vi "Right Front Rocket Backup.vi"() -> (4 "path":cluster{"X":dbl, "Y":dbl}[](array[cluster])=[{"X"=200.0, "Y"=26.0}, {"X"=199.1943498032167, "Y"=26.591866844934284}, {"X"=198.38873809601802, "Y"=27.18374953225293}, {"X"=197.5831805333619, "Y"=27.775644921567796}, {"X"=196.7776935699249, "Y"=28.367551744638334}, {"X"=195.97230663271714, "Y"=28.95947685312332}, {"X"=195.16706591924, "Y"=29.551435458333945}, {"X"=194.36203025886132, "Y"=30.143446988636807}, {"X"=193.5572652684043, "Y"=30.735530675900026}, {"X"=192.75284191693686, "Y"=31.32770409196553}, {"X"=191.9488416559131, "Y"=31.919985289972765}, {"X"=191.1453662297423, "Y"=32.512397057826604}, {"X"=190.34254864947067, "Y"=33.104971168873284}, {"X"=189.54056281731533, "Y"=33.69775128282373}, {"X"=188.73963160206324, "Y"=34.29079446437416}, {"X"=187.94003519101045, "Y"=34.88417230079357}, {"X"=187.14212237118593, "Y"=35.47797290200322}, {"X"=186.34632703384437, "Y"=36.07230473652726}, {"X"=185.5531911950038, "Y"=36.667302723675775}, {"X"=184.76339581382143, "Y"=37.26313582570225}, {"X"=183.97779546937824, "Y"=37.860020685493126}, {"X"=183.1974762909218, "Y"=38.458217383512036}, {"X"=182.42378519481926, "Y"=39.058094370726934}, {"X"=181.65844307990056, "Y"=39.66003129580096}, {"X"=180.90360190480678, "Y"=40.264622933863706}, {"X"=180.16194289999132, "Y"=40.87251655708369}, {"X"=179.43687179220336, "Y"=41.484549595685024}, {"X"=178.73266346217133, "Y"=42.10181051088304}, {"X"=178.05466925868603, "Y"=42.72564542605129}, {"X"=177.40962348032767, "Y"=43.35772858802012}, {"X"=176.80601063295643, "Y"=44.000177475204424}, {"X"=176.25449894606365, "Y"=44.655669174547775}, {"X"=175.76848917552144, "Y"=45.327566980849404}, {"X"=175.36482277513522, "Y"=46.02008856392197}, {"X"=175.0646779497543, "Y"=46.73853223710994}, {"X"=174.86614653066542, "Y"=47.51051459305893}, {"X"=174.7484379619757, "Y"=48.325063754078045}, {"X"=174.6950112849843, "Y"=49.17344929096942}, {"X"=174.6927035694691, "Y"=50.04871852011999}, {"X"=174.73104103819261, "Y"=50.945330054404096}, {"X"=174.80169247736674, "Y"=51.85886492548568}, {"X"=174.89803246459678, "Y"=52.78579710225695}, {"X"=175.01479085792968, "Y"=53.72330893577166}, {"X"=175.14777214158292, "Y"=54.66914161793746}, {"X"=175.293632277303, "Y"=55.621473844165195}, {"X"=175.44970252687955, "Y"=56.578826266134335}, {"X"=175.61385096312907, "Y"=57.53997634478085}, {"X"=175.7843670904187, "Y"=58.5039152993254}, {"X"=175.95989103496223, "Y"=59.469756162119815}, {"X"=176.13929548545426, "Y"=60.43673938057879}, {"X"=176.32170057144518, "Y"=61.404155893682265}, {"X"=176.50635201235707, "Y"=62.37130891959189}, {"X"=176.6926108918171, "Y"=63.33749871042447}, {"X"=176.8799414404591, "Y"=64.30197853375324}, {"X"=177.06786159705038, "Y"=65.26390340878352}, {"X"=177.2559091660838, "Y"=66.2222899350715}, {"X"=177.44363053363736, "Y"=67.17597342387097}, {"X"=177.63056456629263, "Y"=68.12354689215407}, {"X"=177.81621186609976, "Y"=69.06328130793628}, {"X"=178.0, "Y"=69.99303135888502}], 6 "Reverse Path?":bool=TRUE)   [LabVIEW 2018]
uses:
  AutonBuilder/Typedef/Data Point.ctl
panel:
  in  "Data Points":T1[](array[typedef])=[{"X"=200.0, "Y"=26.0, "Theta"=0.0, "Speed %"=0.0, "Disabled?"=FALSE}, {"X"=173.13402061855672, "Y"=45.721254355400696, "Theta"=0.0, "Speed %"=0.0, "Disabled?"=FALSE}, {"X"=178.0, "Y"=69.99303135888502, "Theta"=0.0, "Speed %"=0.0, "Disabled?"=FALSE}]
  out "Graph":cluster{dbl[], dbl[]}[](graph)=[{[180.5, 214.0, 214.0, 180.5, 180.5], [40.25, 40.25, 11.75, 11.75, 40.25]}, {[200.0, 173.13402061855672, 178.0], [26.0, 45.721254355400696, 69.99303135888502]}, {[200.0, 199.1943498032167, 198.38873809601802, 197.5831805333619, 196.7776935699249, 195.97230663271714, 195.16706591924, 194.36203025886132, 193.5572652684043, 192.75284191693686, 191.9488416559131, 191.1453662297423, 190.34254864947067, 189.54056281731533, 188.73963160206324, 187.94003519101045, 187.14212237118593, 186.34632703384437, 185.5531911950038, 184.76339581382143, 183.97779546937824, 183.1974762909218, 182.42378519481926, 181.65844307990056, 180.90360190480678, 180.16194289999132, 179.43687179220336, 178.73266346217133, 178.05466925868603, 177.40962348032767, 176.80601063295643, 176.25449894606365, 175.76848917552144, 175.36482277513522, 175.0646779497543, 174.86614653066542, 174.7484379619757, 174.6950112849843, 174.6927035694691, 174.73104103819261, 174.80169247736674, 174.89803246459678, 175.01479085792968, 175.14777214158292, 175.293632277303, 175.44970252687955, 175.61385096312907, 175.7843670904187, 175.95989103496223, 176.13929548545426, 176.32170057144518, 176.50635201235707, 176.6926108918171, 176.8799414404591, 177.06786159705038, 177.2559091660838, 177.44363053363736, 177.63056456629263, 177.81621186609976, 178.0], [26.0, 26.591866844934284, 27.18374953225293, 27.775644921567796, 28.367551744638334, 28.95947685312332, 29.551435458333945, 30.143446988636807, 30.735530675900026, 31.32770409196553, 31.919985289972765, 32.512397057826604, 33.104971168873284, 33.69775128282373, 34.29079446437416, 34.88417230079357, 35.47797290200322, 36.07230473652726, 36.667302723675775, 37.26313582570225, 37.860020685493126, 38.458217383512036, 39.058094370726934, 39.66003129580096, 40.264622933863706, 40.87251655708369, 41.484549595685024, 42.10181051088304, 42.72564542605129, 43.35772858802012, 44.000177475204424, 44.655669174547775, 45.327566980849404, 46.02008856392197, 46.73853223710994, 47.51051459305893, 48.325063754078045, 49.17344929096942, 50.04871852011999, 50.945330054404096, 51.85886492548568, 52.78579710225695, 53.72330893577166, 54.66914161793746, 55.621473844165195, 56.578826266134335, 57.53997634478085, 58.5039152993254, 59.469756162119815, 60.43673938057879, 61.404155893682265, 62.37130891959189, 63.33749871042447, 64.30197853375324, 65.26390340878352, 66.2222899350715, 67.17597342387097, 68.12354689215407, 69.06328130793628, 69.99303135888502]}, {[201.86128308445547, 207.63107403387954, 206.82587077575548, 206.02079908149562, 205.21589819896602, 204.41136100306696, 203.60742524615034, 202.80427489074197, 202.00202017162016, 201.20075349211936, 200.4006326654585, 199.6019422834876, 198.80511285244344, 198.01070915105655, 197.21941556084556, 196.43204347473875, 195.64957206946087, 194.87321957187837, 194.10453505398385, 193.34550192740312, 192.59866274546755, 191.8671875924176, 191.15535367467203, 190.46779850584568, 189.8119619439668, 189.19520654736073, 188.62851332065927, 188.12564683943538, 187.70339701867377, 187.38310915302534, 187.19128687653216, 187.15842745712516, 187.31454577233842, 187.67602763541524, 188.21336375929673, 188.66707737478282, 188.85194093106554, 188.91683879173272, 188.9426540399829, 188.96803251214928, 189.00926631608758, 189.07168389934404, 189.15554849651394, 189.2589827754278, 189.37937628308103, 189.51403812808726, 189.66047465269054, 189.8165120366586, 189.98025049701062, 190.15019814094478, 190.3249621913328, 190.50352658134514, 190.68498431314302, 190.86852348141622, 191.0534804479116, 191.2392755766644, 191.42534185356658, 191.61111338907307, 191.79602650860252, 191.9794907180509], [11.872079937955483, 38.07595079863937, 38.66753340972582, 39.25907181584417, 39.85054798422794, 40.44184861745318, 41.03284802093431, 41.623473363845285, 42.21371061109062, 42.803560923500925, 43.392985278248176, 43.98187051772098, 44.57002708284787, 45.157206814611015, 45.74312016758301, 46.327436490223526, 46.90976189722709, 47.48959879619045, 48.06629470566628, 48.63898544914682, 49.20652443810576, 49.76744396841678, 50.319631205530676, 50.86082399004236, 51.38683590668063, 51.89352594266694, 52.37382073806938, 52.81789017064861, 53.21204388375076, 53.535748215457176, 53.757663695774845, 53.82991808253255, 53.679278006926594, 53.19621111640238, 52.23166990896362, 51.059712789256025, 50.36312754132175, 50.06906213606161, 50.08628962475435, 50.33658234764442, 50.76007212550217, 51.312669474966135, 51.96220887989153, 52.685147049582135, 53.46408750794995, 54.28601923181995, 55.14104680770596, 56.02169689481024, 56.921811783812096, 57.83729582889918, 58.76385969723334, 59.69893093635797, 60.64009513695385, 61.58498157324474, 62.53169452979284, 63.47857642461773, 64.42383814991307, 65.36551233583458, 66.30152777779178, 67.22963864992576]}, {[198.13871691554453, 190.75762557255388, 189.95160541628056, 189.1455619852282, 188.3394889408838, 187.5332522623673, 186.72670659232966, 185.91978562698068, 185.11251036518846, 184.30493034175436, 183.4970506463677, 182.688790175997, 181.8799844464979, 181.07041648357412, 180.25984764328092, 179.44802690728216, 178.634672672911, 177.81943449581038, 177.00184733602373, 176.18128970023974, 175.35692819328892, 174.527764989426, 173.6922167149665, 172.84908765395545, 171.99524186564676, 171.1286792526219, 170.24523026374746, 169.3396800849073, 168.4059414986983, 167.43613780763, 166.4207343893807, 165.35057043500214, 164.22243257870446, 163.0536179148552, 161.91599214021187, 161.06521568654802, 160.64493499288585, 160.4731837782359, 160.4427530989553, 160.49404956423595, 160.5941186386459, 160.72438102984952, 160.87403321934542, 161.03656150773804, 161.20788827152498, 161.38536692567183, 161.5672272735676, 161.7522221441788, 161.93953157291384, 162.12839282996373, 162.31843895155757, 162.509177443369, 162.7002374704912, 162.891359399502, 163.08224274618917, 163.2725427555032, 163.46191921370814, 163.6500157435122, 163.836397223597, 164.0205092819491], [40.12792006204452, 15.107782891229201, 15.699965654780039, 16.29221802729142, 16.88455550504873, 17.477105088793458, 18.070022895733576, 18.66342061342833, 19.257350740709434, 19.85184726043013, 20.44698530169735, 21.04292359793223, 21.639915254898696, 22.238295751036446, 22.83846876116531, 23.44090811136362, 24.046183906779355, 24.65501067686407, 25.26831074168527, 25.887286202257677, 26.513516932880492, 27.148990798607294, 27.796557535923192, 28.459238601559562, 29.14240996104678, 29.851507171500444, 30.595278453300672, 31.385730851117472, 32.239246968351814, 33.17970896058307, 34.242691254634, 35.481420266563, 36.975855954772214, 38.843966011441566, 41.24539456525627, 43.96131639686183, 46.28699996683434, 48.277836445877234, 50.01114741548563, 51.55407776116377, 52.9576577254692, 54.258924729547765, 55.4844089916518, 56.65313618629279, 57.77886018038044, 58.87163330044872, 59.93890588185573, 60.98613370384056, 62.01770054042753, 63.036182932258406, 64.04445209013119, 65.04368690282581, 66.0349022838951, 67.01897549426175, 67.99611228777421, 68.96600344552527, 69.92810869782888, 70.88158144847355, 71.82503483808078, 72.75642406784428]}, {[], []}, {[], []}, {[], []}, {[], []}, {[], []}]
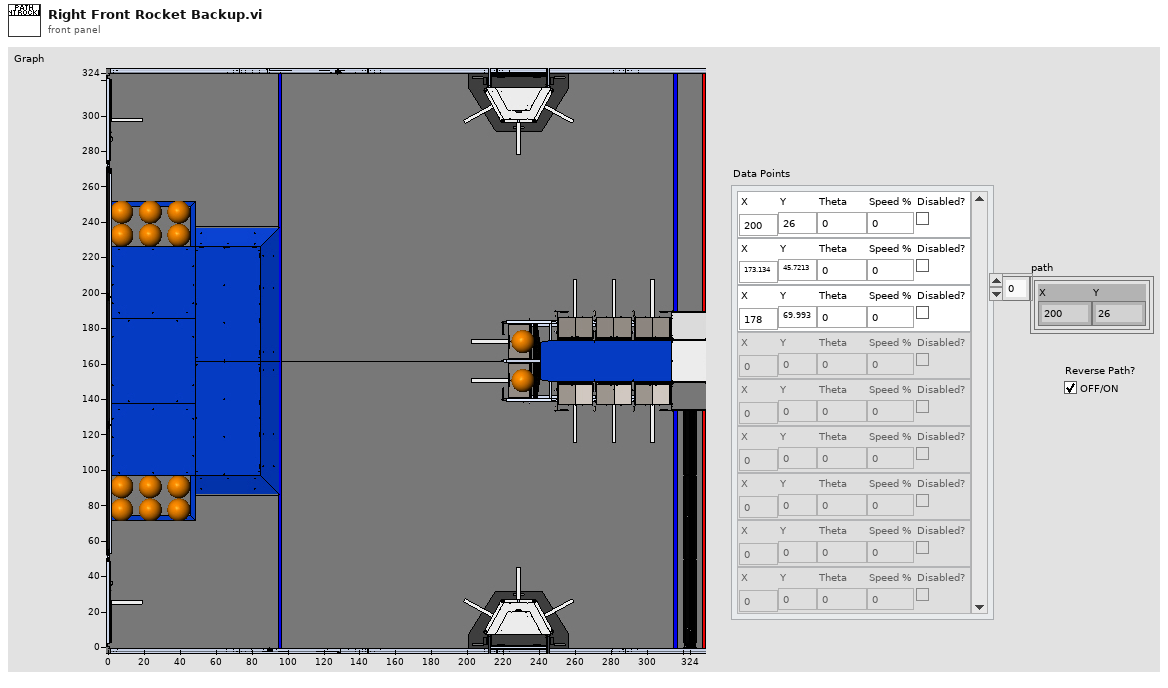
[diagram p1: front panel]
types:
  T1 = typedef "Data Point.ctl" = cluster{"X":dbl, "Y":dbl, "Theta":dbl, "Speed %":dbl, "Disabled?":bool}
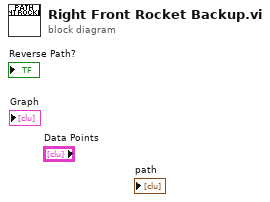
[diagram p0: block diagram]
diagram:
